vi "SWERVE_DRIVE_GET_SPEED_DEMAND.vi"() -> (3 "Drv Chassis Velocity DmD":T1 {"vOmega" format="%10.3f"; "vY" format="%10.3f"; "vX" format="%10.3f"})   [LabVIEW 2019]
uses:
  <vilib>/Rock Robotics/WPI/ThirdParty/JAS_Junk/TrajLib/TypeDef/CHASSIS_SPEEDS.ctl
  SWERVE_DRIVE_GLOBALS.vi
  <vilib>/Rock Robotics/WPI/ThirdParty/JAS_Junk/TrajLib/Trajectory_Library.lvlib
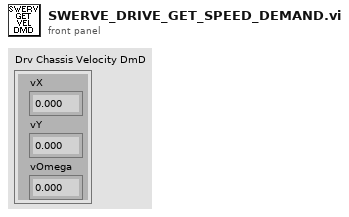
[diagram p1: front panel]
types:
  T1 = typedef "Trajectory_Library.lvlib/CHASSIS_SPEEDS.ctl" = cluster{"vX":dbl, "vY":dbl, "vOmega":dbl}
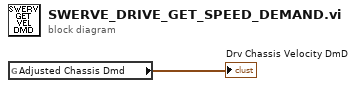
[diagram p0: block diagram]
diagram:
  n1 = global read "SWERVE_DRIVE_GLOBALS.vi" "Adjusted Chassis Dmd"() -> (→"Drv Chassis Velocity DmD":T1)
